vi "Initialize.vi"(8 "error in (no error)":errorcluster) -> (0 "error out":errorcluster, 2 "queue out":refnum<queue>, 3 "Stream Upload Controller out":refnum<class "Stream Upload Controller.lvclass">)   [LabVIEW 2020, in "NI_SFTP.lvlib" / "Stream Upload Controller.lvclass"]
uses:
  <vilib>/net/SFTP/API/Support/Upload/Stream/Stream Upload Controller.lvclass
  <vilib>/net/SFTP/API/Support/Upload/Stream/Stream Upload Controller.lvclass/Stream Upload Controller.ctl
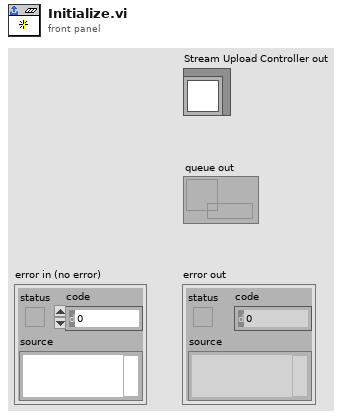
[diagram p1: front panel]
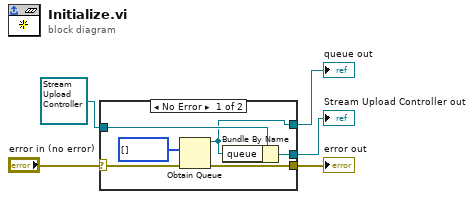
[diagram p0: block diagram]
diagram:
  n1 = case shown="No Error" "error in (no error)" {
    selector: "error in (no error)" -> [w9 w13]
    tunnel: [w8 w13] -> w3
    tunnel: [w11 w12] -> w4
    tunnel: refnum<class "Stream Upload Controller.lvclass"> refnum ("Stream Upload Controller in") -> [w10 w12]
    tunnel: [w7 _] -> w1
    frame No Error {
      n2 = Obtain Queue(element data type=u8[] [] ("data"), error in (no error)=w9) -> (queue out=w7:refnum<queue>, error out=w8:errorcluster)  [unwired: 3 in, 1 out]
      n3 = Bundle By Name(cluster=w10, "queue"=w7) -> (w11:refnum<class "Stream Upload Controller.lvclass">)
    }
    frame Error {
    }
  }
  "error out" <- w3
  "Stream Upload Controller out" <- w4
  "queue out" <- w1
